vi "Hardware_Init.vi"(8 "Error In":errorcluster, 10 "HW Device Name":string, 11 "object in":refnum<class "Hardware.lvclass">) -> (0 "Error Out":errorcluster, 3 "object out":refnum<class "Hardware.lvclass">)   [LabVIEW 2023, in "HAL.lvlib" / "Hardware.lvclass"]
uses:
  Hardware.lvclass
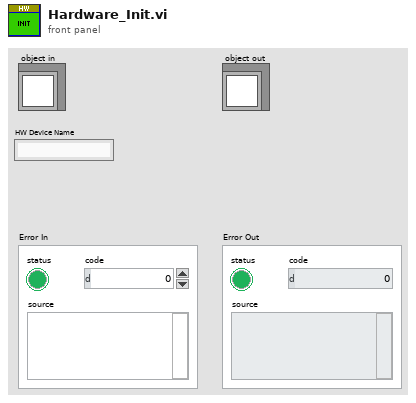
[diagram p1: front panel]
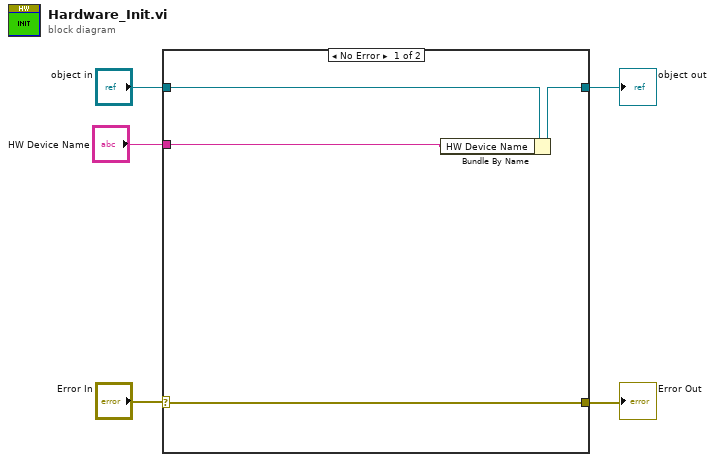
[diagram p0: block diagram]
diagram:
  n1 = case shown="No Error" "Error In" {
    selector: "Error In" -> [w7 w10]
    tunnel: "object in" -> [w9 w11]
    tunnel: [w8 w11] -> w4
    tunnel: [w7 w10] -> w2
    tunnel: "HW Device Name" -> [w6 _]
    frame No Error {
      n2 = Bundle By Name(cluster=w9, "HW Device Name"=w6) -> (w8:refnum<class "Hardware.lvclass">)
    }
    frame Error {
    }
  }
  "object out" <- w4
  "Error Out" <- w2
